vi "LIst Searcheable Folders.vi"() -> (3 "Searcheable Folders":path[](array[path]))   [LabVIEW 2020, in "Caraya.lvlib" / "Basic Test Manager.lvclass"]
uses:
  Basic Test Manager.lvclass
  <userlib>/_OpenG.lib/file/file.llb/File Exists - Scalar__ogtk.vi
  <userlib>/_OpenG.lib/array/array.llb/Remove Duplicates from 1D Array (Path)__ogtk.vi
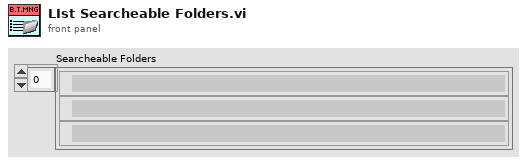
[diagram p1: front panel]
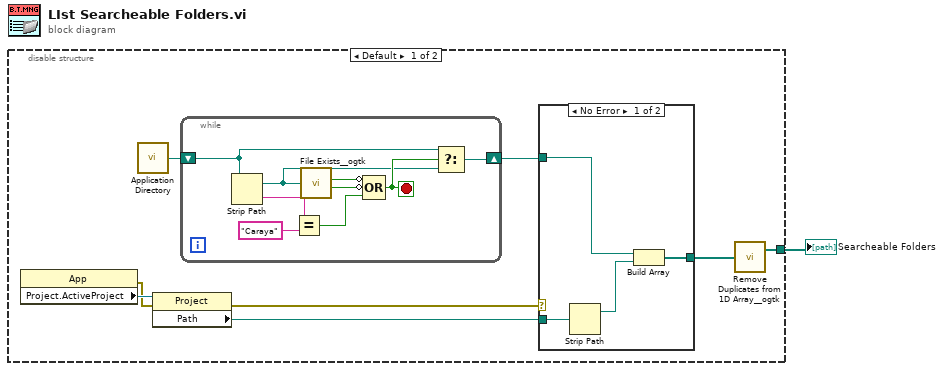
[diagram p0: block diagram]
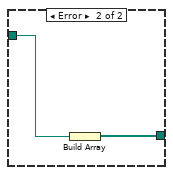
[diagram p2: hidden frame]
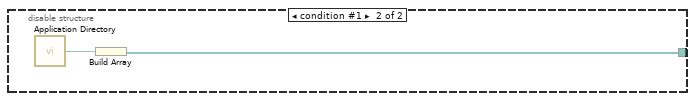
[diagram p3: hidden frame]
diagram:
  n1 = disable-structure shown="Default" {
    disable-tunnel: [w5 w25] -> w1
    frame condition #0 (active) {
      n2 = property class="App"() -> (error out=w7:errorcluster, "Project.ActiveProject"=w9:refnum<vi>)  [unwired: 2 in, 1 out]
      n3 = call <vilib>:"Application Directory.vi"() -> ("Application Directory"=w3:path)
      n4 = property class="Project"(reference=w9, error in=w7) -> (error out=w4:errorcluster, "Path"=w8:path)  [unwired: 1 out]
      n5 = while {
        shift-right: [w10] -> w2
        shift-left: w3 -> [w12]
        stop <- w13 stop-if-true
        n6 = Strip Path(path=w12) -> (stripped path=w11:path, name=w18:string)
        n7 = Equal?(x=w18, y="Caraya") -> (x = y?=w14:bool)
        n8 = call-poly <userlib>:"File Exists__ogtk.vi"("file path"=w11) -> ("is directory"=w16:bool, "exists"=w15:bool)  [unwired: 6 in]
        n9 = Compound Arithmetic op=OR(invert w16, invert w15, w14) -> (w13:bool)
        n10 = Select(t=w12, s=w13, f=w11) -> (s? t:f=w10:path)
      }
      n11 = case shown="No Error" w4 {
        tunnel: w8 -> [w22 _]
        tunnel: w2 -> [w21 w24]
        tunnel: [w20 w23] -> w6
        frame No Error {
          n12 = Strip Path(path=w22) -> (stripped path=w19:path)  [unwired: 1 out]
          n13 = Build Array(w21, w19) -> (w20:path[])
        }
        frame Error {
          n14 = Build Array(w24) -> (w23:path[])
        }
      }
      n15 = call-poly <userlib>:"Remove Duplicates from 1D Array__ogtk.vi"("Input Array"=w6) -> ("Output Array"=w5:path[])  [unwired: 1 out]
    }
    frame condition #1 {
      n16 = call <vilib>:"Application Directory.vi"() -> ("Application Directory"=w26:path)
      n17 = Build Array(w26) -> (w25:path[])
    }
  }
  "Searcheable Folders" <- w1
